vi "FormatDataFromFpga.vi"(11 "Raw data":u64[](array[numeric])) -> (3 "Scaled":dbl[][](array[numeric]))   [LabVIEW 2025]
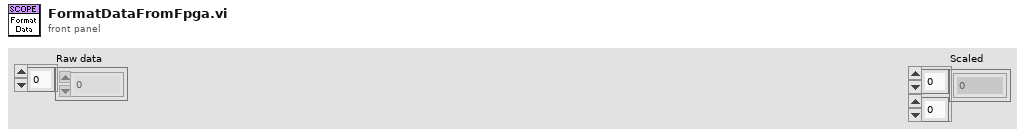
[diagram p1: front panel]
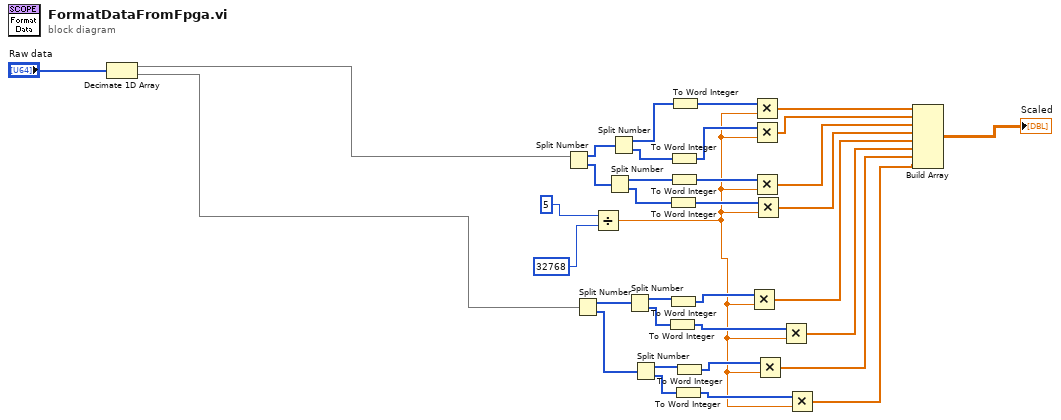
[diagram p0: block diagram]
diagram:
  n1 = Decimate 1D Array("Raw data") -> (w12:u64[], w11:u64[])
  n2 = Split Number(x=w12) -> (hi(x)=w32:u32[], lo(x)=w28:u32[])
  n3 = Split Number(x=w11) -> (hi(x)=w17:u32[], lo(x)=w4:u32[])
  n4 = Divide(x=5, y=32768) -> (x/y=w3:dbl)
  n5 = Split Number(x=w28) -> (hi(x)=w30:u16[], lo(x)=w31:u16[])
  n6 = Split Number(x=w32) -> (hi(x)=w33:u16[], lo(x)=w29:u16[])
  n7 = Split Number(x=w17) -> (hi(x)=w16:u16[], lo(x)=w15:u16[])
  n8 = Split Number(x=w4) -> (hi(x)=w5:u16[], lo(x)=w6:u16[])
  n9 = To Word Integer(number=w15) -> (16bit integer=w13:i16[])
  n10 = To Word Integer(number=w31) -> (16bit integer=w23:i16[])
  n11 = To Word Integer(number=w16) -> (16bit integer=w14:i16[])
  n12 = To Word Integer(number=w29) -> (16bit integer=w25:i16[])
  n13 = To Word Integer(number=w30) -> (16bit integer=w24:i16[])
  n14 = To Word Integer(number=w33) -> (16bit integer=w27:i16[])
  n15 = To Word Integer(number=w6) -> (16bit integer=w8:i16[])
  n16 = To Word Integer(number=w5) -> (16bit integer=w7:i16[])
  n17 = Multiply(x=w14, y=w3) -> (x*y=w18:dbl[])
  n18 = Multiply(x=w27, y=w3) -> (x*y=w26:dbl[])
  n19 = Multiply(x=w25, y=w3) -> (x*y=w22:dbl[])
  n20 = Multiply(x=w24, y=w3) -> (x*y=w21:dbl[])
  n21 = Multiply(x=w23, y=w3) -> (x*y=w20:dbl[])
  n22 = Multiply(x=w7, y=w3) -> (x*y=w2:dbl[])
  n23 = Multiply(x=w13, y=w3) -> (x*y=w19:dbl[])
  n24 = Multiply(x=w8, y=w3) -> (x*y=w1:dbl[])
  n25 = Build Array(w26, w22, w21, w20, w18, w19, w2, w1) -> (→"Scaled":dbl[][])
